vi "Tabelle faerben.vi"(8 "error in (no error)":errorcluster caption="Fehler (Eingang, kein Fehler)", 11 "Ergebnisse":refnum<vi>) -> (0 "error out":errorcluster caption="Fehler (Ausgang)")   [LabVIEW 2015, in "Schedule Modul.lvlib"]
uses:
  Schedule Modul.lvlib
  Ergebnis Tabelle.ctl
  <vilib>/Utility/miscctls.llb/LVRowAndColumnTypeDef.ctl
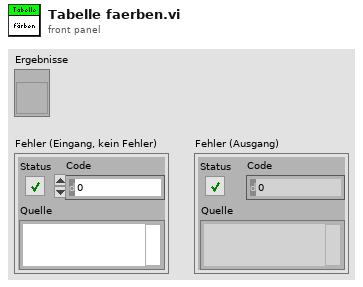
[diagram p1: front panel]
types:
  T1 = typedef "LVRowAndColumnTypeDef.ctl" = cluster{"Row":i32, "Column":i32}
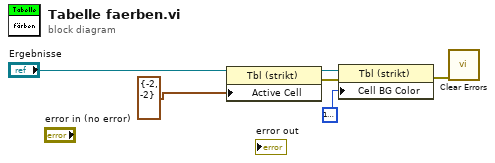
[diagram p0: block diagram]
diagram:
  n1 = property class="Tbl (strikt)"(reference="Ergebnisse", "Active Cell"=T1 {"Row"=-2, "Column"=-2} ("Aktive Zelle:Aktive Zelle")) -> (reference out=w5:refnum<vi>, error out=w4:errorcluster)  [unwired: 1 in]
  n2 = property class="Tbl (strikt)"(reference=w5, error in=w4, "Cell BG Color"=u32 16777225) -> (error out=w3:errorcluster)  [unwired: 1 out]
  n3 = call <vilib>:"Clear Errors.vi"("error in (no error)"=w3) -> ()  [unwired: 5 in, 2 out]
